vi "2D Dbl to ITX Wave.vi"(1 "2D Array":dbl[][](array[numeric]), 2 "Wavename":string) -> (0 "ITX Wave":string)   [LabVIEW 2016, in "LV-Data.ITX.lvclass"]
uses:
  LV-Data.ITX.lvclass
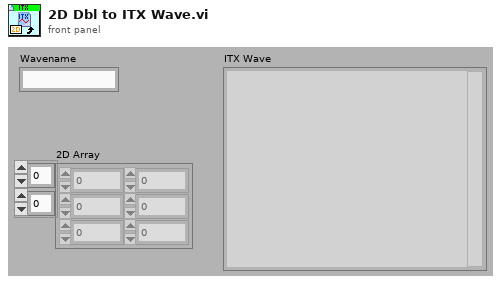
[diagram p1: front panel]
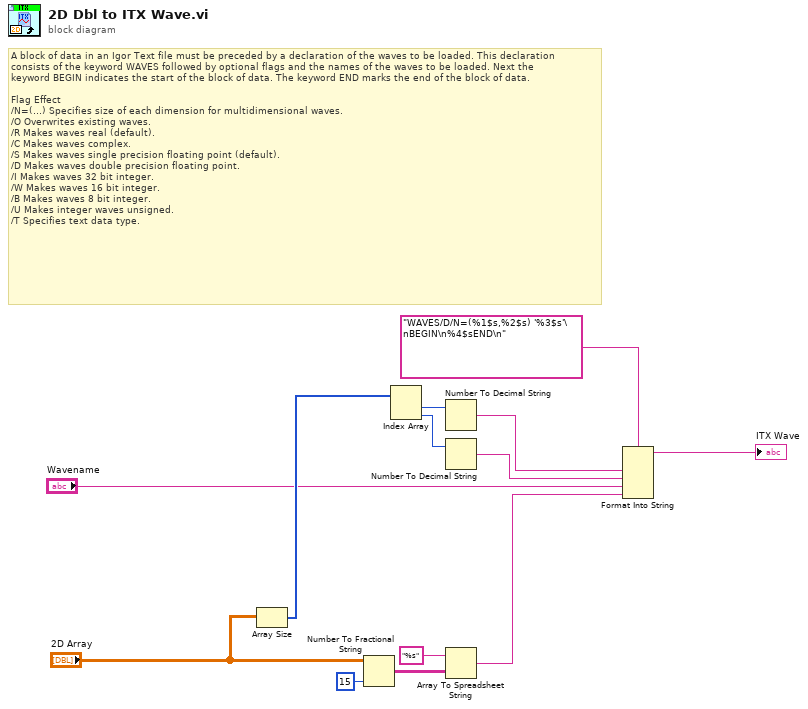
[diagram p0: block diagram]
diagram:
  # "A block of data in an Igor Text file must be preceded by a declaration of the waves to be loaded. This declaration\nconsists of the keyword WAVES followed by optional flags and the names of the waves to be loaded. Next the\nkeyword BEGIN indicates the start of the block of data. The keyword END marks the end of the block of data.\n\nFlag Effect\n/N=(…) Specifies size of each dimension for multidimensional waves.\n/O Overwrites existing waves.\n/R Makes waves real (default).\n/C Makes waves complex.\n/S Makes waves single precision floating point (default).\n/D Makes waves double precision floating point.\n/I Makes waves 32 bit integer.\n/W Makes waves 16 bit integer.\n/B Makes waves 8 bit integer.\n/U Makes integer waves unsigned.\n/T Specifies text data type."
  n1 = Array Size(array="2D Array") -> (size(s)=w11:i32[])
  n2 = Number To Fractional String(number="2D Array", precision (6)=i16 15) -> (F-format string=w8:string[][])  [unwired: 2 out]
  n3 = Index Array(array=w11) -> (element #1=w12:i32, element #2=w13:i32)  [unwired: 2 in]
  n4 = Number To Decimal String(number=w12) -> (decimal integer string=w2:string)  [unwired: 1 out]
  n5 = Number To Decimal String(number=w13) -> (decimal integer string=w4:string)  [unwired: 1 out]
  n6 = Array To Spreadsheet String(array=w8, 3:"%s" ("format string")) -> (spreadsheet string=w1:string)  [unwired: 1 out]
  n7 = Format Into String(format string="WAVES/D/N=(%1$s,%2$s) '%3$s'\nBEGIN\n%4$sEND\n", w2, w4, "Wavename", w1) -> (resulting string=→"ITX Wave":string)  [unwired: 2 in, 1 out]
